vi "Add Team.vi"(8 "error in (no error)":errorcluster, 10 "Team":refnum<class "Team.lvclass">, 11 "Game Config Panel in":refnum<class "Game Config Panel.lvclass">) -> (0 "error out":errorcluster, 3 "Game Config Panel out":refnum<class "Game Config Panel.lvclass">)   [LabVIEW 2020, in "SB App.lvlib" / "Game Config Panel.lvclass"]
uses:
  Game Config Panel.lvclass
  SquareBattle/Team/Team.lvclass
  Add Team Data.ctl
  Game Config Panel.lvclass/Game Config Panel.ctl
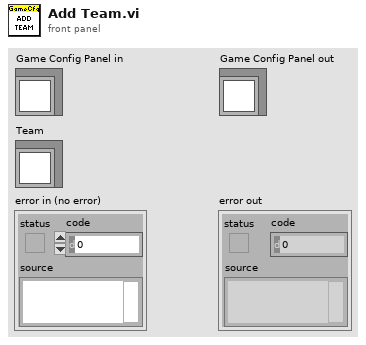
[diagram p1: front panel]
types:
  T1 = typedef "SB App.lvlib/Game Config Panel.lvclass/Add Team Data.ctl" = cluster{"Team":refnum<class "Team.lvclass">}
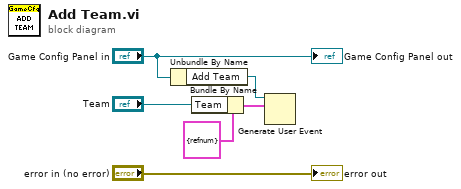
[diagram p0: block diagram]
diagram:
  n1 = Unbundle By Name("Game Config Panel in") -> ("Add Team"=w4:refnum<user-event>)
  n2 = Bundle By Name(cluster=T1 {"Team"=refnum} ("event data"), "Team"="Team") -> (w2:T1)
  n3 = Generate User Event(user event=w4, event data cluster=w2) -> ()  [unwired: 2 in, 2 out]
  "error out" <- "error in (no error)"
  "Game Config Panel out" <- "Game Config Panel in"
